vi "Auto Align.vi"(0 "Auto Aim":bool, 1 "Left Axis":dbl, 2 "Right Axis":dbl, 4 "reinitialize? (F)":bool) -> (8 "Left Axis":dbl, 9 "Right Axis":dbl)   [LabVIEW 2016]
uses:
  Robot Global Data.vi
  <vilib>/Analysis/NI_AALPro.lvlib
  <vilib>/Analysis/_algsub.llb/Real Vector Norm.vi
  <vilib>/Analysis/_algsub.llb/Vector Norm Type.ctl
panel:
  in  "PID Gains Angle Close":cluster{"Kp":dbl, "Ki":dbl, "Kd":dbl}={"Kp"=0.015, "Ki"=0.0, "Kd"=0.005}
  in  "PID Gains v":cluster{"Kp":dbl, "Ki":dbl, "Kd":dbl}={"Kp"=0.01, "Ki"=0.0, "Kd"=0.0}
  in  "V ff":dbl=-1.0
  in  "Alpha":dbl=0.5
  in  "Dead Distance":dbl=100.0
  in  "Theta f":dbl
  in  "ff comp":dbl=1.0
  in  "PID Gains Angle Far":cluster{"Kp":dbl, "Ki":dbl, "Kd":dbl}={"Kp"=0.015, "Ki"=0.0, "Kd"=0.005}
  out "Angle Error":dbl(graph)
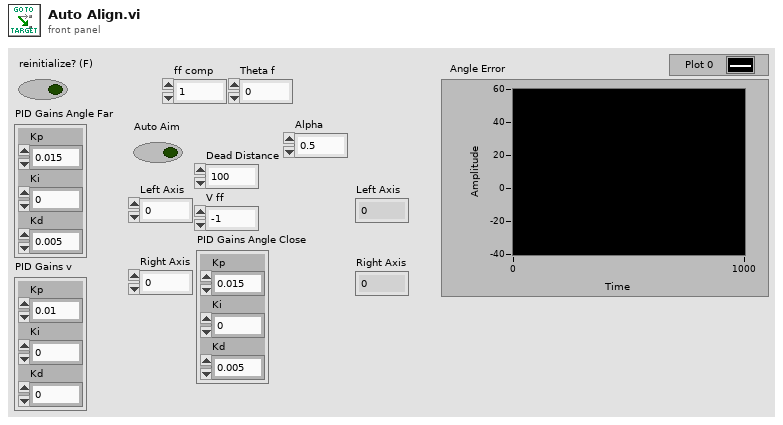
[diagram p1: front panel]
types:
  T1 = typedef "NI_AALPro.lvlib/Vector Norm Type.ctl" = u16
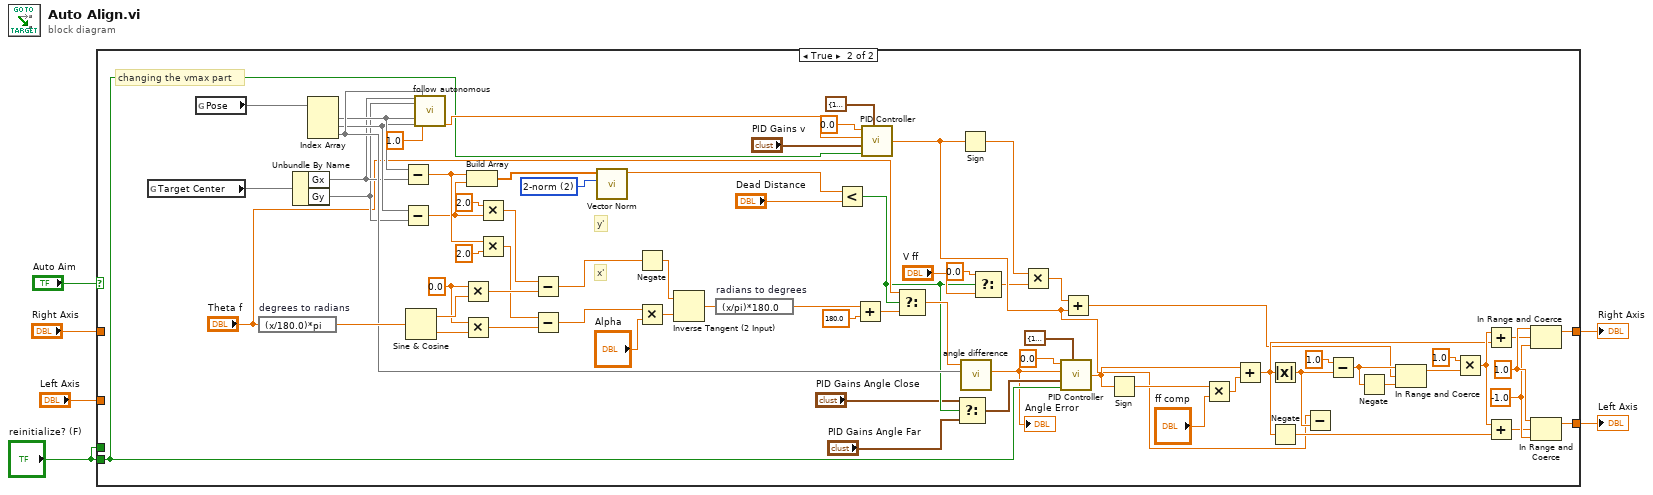
[diagram p0: block diagram]
diagram:
  n1 = case shown="True" "Auto Aim" {
    tunnel: [w7 w81] -> w3
    tunnel: [w8 w80] -> w2
    tunnel: "Right Axis" -> [w8 _]
    tunnel: "Left Axis" -> [w7 _]
    tunnel: "reinitialize? (F)" -> [_ w18]
    tunnel: "reinitialize? (F)" -> [_ _]
    frame False {
    }
    frame True {
      w61 = 0.0 ("K")
      w41 = T1 2 items=["1-norm"=1, "2-norm"=2, "Inf-norm"=3, "-Inf-norm"=4, "User Defined"=5] ("norm type")
      w78 = -1.0 ("upper limit")
      w79 = 1.0 ("upper limit")
      # "changing the vmax part"
      # "x'"
      # "y'"
      n2 = global read "Robot Global Data.vi" "Target Center"() -> (w66)
      n3 = global read "Robot Global Data.vi" "Pose"() -> (w45)
      n4 = expression code="(x/180.0)*pi" "degrees to radians"("Theta f") -> (w63:dbl)
      n5 = Unbundle By Name(w66) -> ("Gx"=w48, "Gy"=w47)
      n6 = Index Array(array=w45) -> (element #1=w50, element #2=w49, element #3=w51)  [unwired: 3 in]
      n7 = Subtract(x=w50, y=w48) -> (x-y=w44:dbl)
      n8 = Subtract(x=w49, y=w47) -> (x-y=w43:dbl)
      n9 = Sine & Cosine(0:w63) -> (1:w62:dbl, 2:w60:dbl)
      n10 = call "follow autonomous.vi"("x"=w48, "y"=w47, "robot x"=w50, "robot y"=w49, "robot angle"=w51, "speed kp"=1.0) -> ("newV"=w21:dbl)  [unwired: 13 in]
      n11 = Multiply(x=w61, y=w62) -> (x*y=w58:dbl)
      n12 = Multiply(x=w61, y=w60) -> (x*y=w56:dbl)
      n13 = Build Array(w44, w43) -> (w42:dbl[])
      n14 = Multiply(x=2.0, y=w43) -> (x*y=w59:dbl)
      n15 = Multiply(x=w44, y=2.0) -> (x*y=w57:dbl)
      n16 = Subtract(x=w59, y=w58) -> (x-y=w29:dbl)
      n17 = Subtract(x=w57, y=w56) -> (x-y=w28:dbl)
      n18 = call-poly <vilib>:"Vector Norm.vi"("norm type"=w41, "Input Vector"=w42) -> ("norm"=w40:dbl)  [unwired: 8 in, 1 out]
      n19 = Negate(x=w29) -> (-x=w52:dbl)
      n20 = Multiply(x=w28, y="Alpha") -> (x*y=w27:dbl)
      n21 = Inverse Tangent (2 Input)(1:w27, 2:w52) -> (0:w55:dbl)
      n22 = expression code="(x/pi)*180.0" "radians to degrees"(w55) -> (w54:dbl)
      n23 = Less?(x=w40, y="Dead Distance") -> (x < y?=w13:bool)
      n24 = Add(x=w54, y=180.0) -> (x+y=w37:dbl)
      n25 = call "PID Controller.vi"("setpoint"=0.0, "process variable"=w21, "PID Gains"="PID Gains v", "Reinitialize Integral"=w18, "Constrain"=cluster{"Max Control":dbl, "Min Control":dbl} {"Max Control"=1.0, "Min Control"=-1.0}) -> ("Control Signal"=w20:dbl)
      n26 = Select(t="Theta f", s=w13, f=w37) -> (s? t:f=w35:dbl)
      n27 = Select(t="PID Gains Angle Close", s=w13, f="PID Gains Angle Far") -> (s? t:f=w11:cluster{"Kp":dbl, "Ki":dbl, "Kd":dbl})
      n28 = Sign(1:w20) -> (0:w26:dbl)
      n29 = call "angle difference.vi"("angle2"=w51, "angle1"=w35) -> ("angle diff"=w9:dbl)  [unwired: 9 in]
      "Angle Error" <- w9
      n30 = Select(t=0.0, s=w13, f="V ff") -> (s? t:f=w15:dbl)
      n31 = Multiply(x=w26, y=w15) -> (x*y=w25:dbl)
      n32 = call "PID Controller.vi"("setpoint"=0.0, "process variable"=w9, "PID Gains"=w11, "Reinitialize Integral"=w18, "Constrain"=cluster{"output high":dbl, "output low":dbl} {"output high"=1.0, "output low"=-1.0} ("output range")) -> ("Control Signal"=w67:dbl)
      n33 = Add(x=w25, y=w20) -> (x+y=w24:dbl)
      n34 = Sign(1:w67) -> (0:w69:dbl)
      n35 = Multiply(x=w69, y="ff comp") -> (x*y=w68:dbl)
      n36 = Add(x=w67, y=w68) -> (x+y=w38:dbl)
      n37 = Absolute Value(x=w38) -> (abs(x)=w33:dbl)
      n38 = Negate(x=w38) -> (-x=w74:dbl)
      n39 = Subtract(x=w20, y=w33) -> ()  [unwired: 1 out]
      n40 = Subtract(x=1.0, y=w33) -> (x-y=w32:dbl)
      n41 = Negate(x=w32) -> (-x=w31:dbl)
      n42 = In Range and Coerce(upper limit=w32, x=w24, lower limit=w31) -> (coerced(x)=w72:dbl)  [unwired: 1 out]
      n43 = Multiply(x=1.0, y=w72) -> (x*y=w71:dbl)
      n44 = Add(x=w71, y=w38) -> (x+y=w75:dbl)
      n45 = Add(x=w71, y=w74) -> (x+y=w73:dbl)
      n46 = In Range and Coerce(upper limit=w79, x=w75, lower limit=w78) -> (coerced(x)=w80:dbl)  [unwired: 1 out]
      n47 = In Range and Coerce(upper limit=w79, x=w73, lower limit=w78) -> (coerced(x)=w81:dbl)  [unwired: 1 out]
    }
  }
  "Left Axis" <- w3
  "Right Axis" <- w2
